vi "from_json.vi"(8 "error in":errorcluster, 10 "dataset JSON":string, 11 "Client":refnum<class "Nominal Client.lvclass">) -> (0 "error out":errorcluster, 3 "Dataset":refnum<class "dataset.lvclass">)   [LabVIEW 2020, in "datasources.lvlib" / "dataset.lvclass"]
uses:
  dataset.lvclass
  Nominal Client/Nominal Client.lvclass
  dataset.lvclass/dataset.ctl
  9732f3ad-4379-4d2e-b429-3f31743c0da7.vi
  70fcde8b-cfa6-496f-aa5e-b47ccf35a795.vi
  97724406-c35b-4f72-914b-b01749b4f1b5.vi
  rid.set.vi
  datasetName.set.vi
  datasetDescription.set.vi
  object.set.vi
  <vilib>/JDP Science/JSONtext/Find Item.vi
  <vilib>/JDP Science/JSONtext/Next JSON Value.vi
  <vilib>/JDP Science/JSONtext/String Subset.vi
  <vilib>/JDP Science/JSONtext/Parsing/Advance past next JSON Value (inlined COPY).vi
  <vilib>/JDP Science/JSONtext/Parsing/Advance past whitespace.vi
  <vilib>/JDP Science/JSONtext/Parsing/Advance past String.vi
  <vilib>/JDP Science/JSONtext/Parsing/Advance past Number.vi
  <vilib>/JDP Science/JSONtext/Parsing/Advance past Line Ending.vi
  <vilib>/JDP Science/JSONtext/Parsing/Parse Full Path or Item Name.vi
  <vilib>/JDP Science/JSONtext/Parsing/Advance past Array.vi
  <vilib>/JDP Science/JSONtext/Parsing/Advance past Object.vi
  <vilib>/JDP Science/JSONtext/support/Error Cluster From Code.vi
  <vilib>/JDP Science/JSONtext/Offset/Find Item Locations by Path.vi
  <vilib>/JDP Science/JSONtext/JSON text to Variant.vi
  <vilib>/JDP Science/JSONtext/LVClass Serializer/JSONtext LVClass Serializer.lvclass
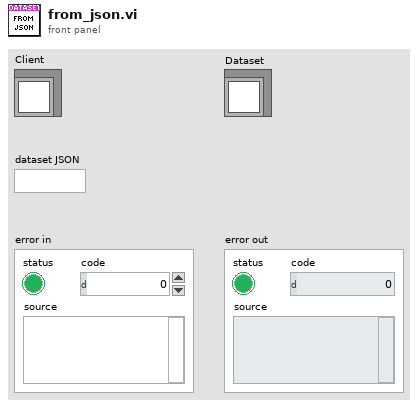
[diagram p1: front panel]
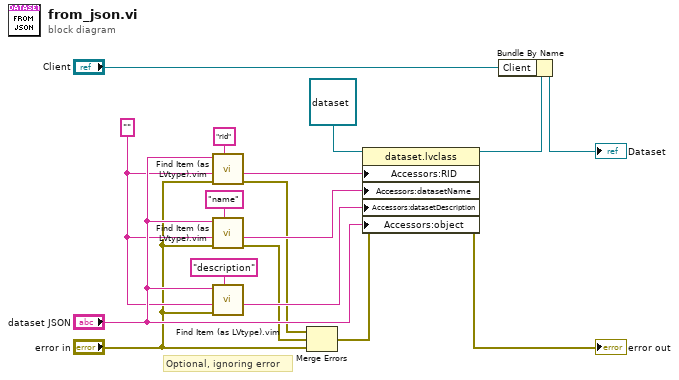
[diagram p0: block diagram]
diagram:
  w11 = "" ("$Path or Item Name")
  # "Optional, ignoring error"
  n1 = call "Find Item (as LVtype).vim"("$Path or Item Name"="rid", "error in (no error)"="error in", "Data Type and Default Value"=w11, "JSON"="dataset JSON") -> ("error out"=w7:errorcluster, "Data"=w10:string)  [unwired: 4 in, 2 out]
  n2 = call "Find Item (as LVtype).vim"("$Path or Item Name"="name", "error in (no error)"="error in", "Data Type and Default Value"=w11, "JSON"="dataset JSON") -> ("error out"=w6:errorcluster, "Data"=w9:string)  [unwired: 4 in, 2 out]
  n3 = call "Find Item (as LVtype).vim"("$Path or Item Name"="description", "error in (no error)"="error in", "Data Type and Default Value"=w11, "JSON"="dataset JSON") -> ("Data"=w8:string)  [unwired: 4 in, 3 out]
  n4 = Merge Errors(w7, w6, "error in") -> (w4:errorcluster)
  n5 = property class="dataset.lvclass"(reference=refnum<class "dataset.lvclass"> refnum ("Dataset"), error in=w4, "Accessors:RID"=w10, "Accessors:datasetName"=w9, "Accessors:datasetDescription"=w8, "Accessors:object"="dataset JSON") -> (reference out=w3:refnum<class "dataset.lvclass">, error out=→"error out":errorcluster)
  n6 = Bundle By Name(cluster=w3, "Client"="Client") -> (→"Dataset":refnum<class "dataset.lvclass">)
